vi "Wait.vi"(10 "milliseconds to wait":u32, 11 "Execute?":bool) -> (3 "Done":bool)   [LabVIEW 2012]
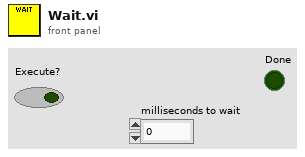
[diagram p1: front panel]
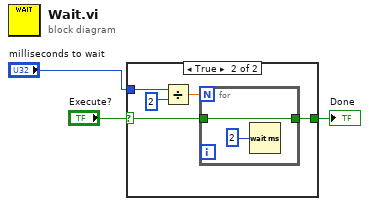
[diagram p0: block diagram]
diagram:
  n1 = case shown="True" "Execute?" {
    selector: "Execute?" -> [w4 w6]
    tunnel: [w4 w5] -> w2
    tunnel: "milliseconds to wait" -> [_ w9]
    frame False {
    }
    frame True {
      n2 = Divide(x=w9, y=u32 2) -> (x/y=w7:dbl)
      n3 = for {
        N: w7 -> [_]
        tunnel: w6 -> [w10]
        tunnel: [w10] -> w5
        n4 = Wait (ms)(milliseconds to wait=u32 2) -> ()  [unwired: 1 out]
      }
    }
  }
  "Done" <- w2
